vi "17-ySteps&PositionToVelocity.vi"(10 "y":i32, 11 "n":i32) -> (3 "vy":dbl)   [LabVIEW 2019, in "17.lvlib"]
uses:
  17.lvlib
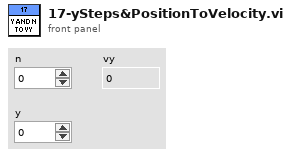
[diagram p1: front panel]
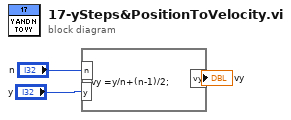
[diagram p0: block diagram]
diagram:
  n1 = formula code="vy =y/n+(n-1)/2;"("n"="n", "y"="y") -> ("vy"=→"vy":dbl)
